vi "Elevator_Test.vi"(0 "Left_Joystick_Press":bool, 1 "LB_Press":bool, 2 "A_Button":bool, 3 "Left_Joystick_Y":dbl) -> ()   [LabVIEW 2018]
uses:
  Subsytems/Elevator/Elevator_Notifier.ctl
  Subsytems/Elevator/Elevator_Control_Type.ctl
  Subsytems/Elevator/Elevator_Enum_States.ctl
  Global_Variables/Elevator_Globals.vi
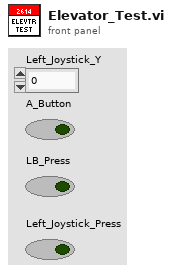
[diagram p1: front panel]
types:
  T1 = typedef "Elevator_Notifier.ctl" = cluster{"Elevator_Control_Type":T2, "Shift":bool, "Brake":bool, "Manual_Lift_Up":bool, "Manual_Lift_Down":bool, "Climb_Advance":bool, "Climb_Reverse":bool, "Low_Rocket":bool, "Mid_Rocket":bool, "High_Rocket":bool, "Cargo_Ship":bool, "Hatch_Floor":bool, "Cargo_Floor":bool, "HP_Hatch":bool, "HP_Cargo":bool, "Depot_Cargo":bool, "Stow":bool, "Set_Position":T3, "Intake_Mode":bool, "Climb_Distance":dbl, "Level_Two":bool, "Parameter_One":dbl, "Parameter_Two":dbl, "Parameter_Three":dbl, "Step":i32, "Elevator_Notifier":refnum<notifier>, "Brake_State":bool, "Shift_State":bool}
  T2 = typedef "Elevator_Control_Type.ctl" = enum16{"No_Op", "Shift", "Brake", "Manual_Elevator_Up", "Manual_Elevator_Down", "Manual_Climb_Up", "Manual_Climb_Down", "Manual_Position_Control", "Elevator_Retract", "Elevator_Extend", "Brake_In_Climb", "Position_Control", "Position"}
  T3 = typedef "Elevator_Enum_States.ctl" = enum16{"Current_Position", "High_Rocket_Hatch_Panel_Floor", "High_Rocket_Hatch_Panel", "Mid_Rocket_Hatch_Panel_Floor", "Mid_Rocket_Hatch_Panel", "Low_Rocket_Hatch_Panel", "Cargo_Ship_Hatch_Panel", "Loading_Station_Hatch_Panel", "Ground_Pickup_Hatch_Panel", "High_Rocket_Cargo", "Mid_Rocket_Cargo", "Low_Rocket_Cargo", "Cargo_Ship_Cargo", "Loading_Station_Cargo", "Ground_Pickup_Cargo", "Depot_Pickup_Cargo", "Stow_Cargo"}
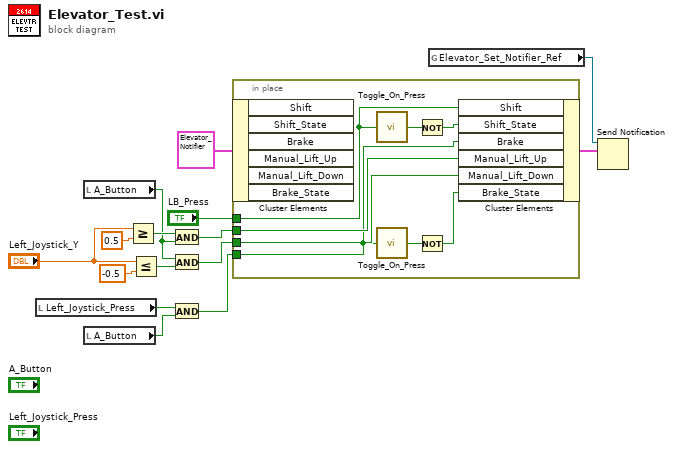
[diagram p0: block diagram]
diagram:
  n1 = local read "Left_Joystick_Press"() -> (w2:bool)
  n2 = local read "A_Button"() -> (w7:bool)
  n3 = local read "A_Button"() -> (w3:bool)
  n4 = Greater Or Equal?(x="Left_Joystick_Y", y=0.5) -> (x >= y?=w8:bool)
  n5 = Less Or Equal?(x="Left_Joystick_Y", y=-0.5) -> (x <= y?=w9:bool)
  n6 = And(x=w8, y=w7) -> (x .and. y?=w6:bool)
  n7 = And(x=w7, y=w9) -> (x .and. y?=w5:bool)
  n8 = And(x=w2, y=w3) -> (x .and. y?=w1:bool)
  n9 = in-place {
    in-place-border: w6 -> [w23]
    in-place-border: w5 -> [w22]
    in-place-border: "LB_Press" -> [w20]
    in-place-border: w1 -> [w19]
    n10 = in-place-cluster #1(T1 {"Elevator_Control_Type"=enum."No_Op", "Shift"=FALSE, "Brake"=FALSE, "Manual_Lift_Up"=FALSE, "Manual_Lift_Down"=FALSE, "Climb_Advance"=FALSE, "Climb_Reverse"=FALSE, "Low_Rocket"=FALSE, "Mid_Rocket"=FALSE, "High_Rocket"=FALSE, "Cargo_Ship"=FALSE, "Hatch_Floor"=FALSE, "Cargo_Floor"=FALSE, "HP_Hatch"=FALSE, "HP_Cargo"=FALSE, "Depot_Cargo"=FALSE, "Stow"=FALSE, "Set_Position"=enum."High_Rocket_Hatch_Panel", "Intake_Mode"=FALSE, "Climb_Distance"=0.0, "Level_Two"=FALSE, "Parameter_One"=0.0, "Parameter_Two"=0.0, "Parameter_Three"=0.0, "Step"=0, "Elevator_Notifier"=refnum, "Brake_State"=FALSE, "Shift_State"=FALSE} ("Elevator_Notifier")) -> ()  [unwired: 6 out]
    n11 = call "Toggle_On_Press.vi"("Boolean"=w20) -> ("Boolean Out"=w21:bool)
    n12 = call "Toggle_On_Press.vi"("Boolean"=w19) -> ("Boolean Out"=w18:bool)
    n13 = Not(x=w21) -> (.not. x?=w16:bool)
    n14 = Not(x=w18) -> (.not. x?=w17:bool)
    n15 = in-place-cluster #1("Shift"=w20, "Shift_State"=w16, "Brake"=w19, "Manual_Lift_Up"=w23, "Manual_Lift_Down"=w22, "Brake_State"=w17) -> (w15:T1)
  }
  n16 = global read "Elevator_Globals.vi" "Elevator_Set_Notifier_Ref"() -> (w14:refnum<notifier>)
  n17 = Send Notification(notification=w15, notifier=w14) -> ()  [unwired: 1 in, 2 out]
